vi "Read.vi"(7 "Read Type":T1, 8 "error in (no error)":errorcluster, 11 "NetworkStreamReader in":refnum<class "NetworkStreamReader.lvclass">) -> (0 "error out":errorcluster, 2 "element":variant, 3 "NetworkStreamReader out":refnum<class "NetworkStreamReader.lvclass">)   [LabVIEW 2011, in "NetworkStreamReader.lvclass"]
doc: "Returns the requested value (either the next element available in the buffer or the most recent element). If there are no elements available in the queue, this VI will return the last valid value it returned."
uses:
  NetworkStreamReader.lvclass
  readType.ctl
  NetworkStreamReader.lvclass/NetworkStreamReader.ctl
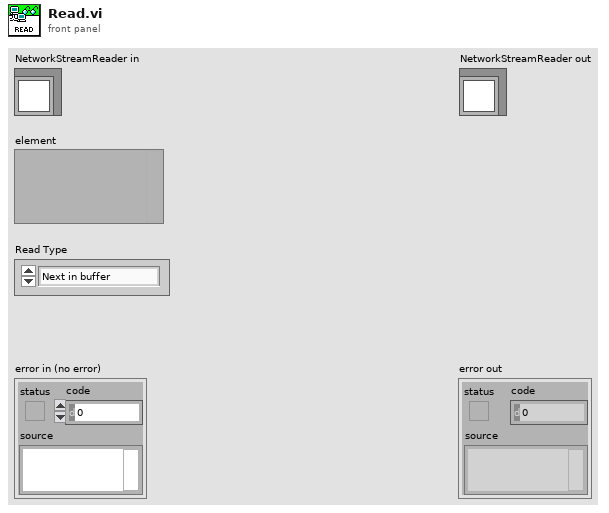
[diagram p1: front panel]
types:
  T1 = typedef "NetworkStreamReader.lvclass/readType.ctl" = enum16{"Next in buffer", "Most current"}
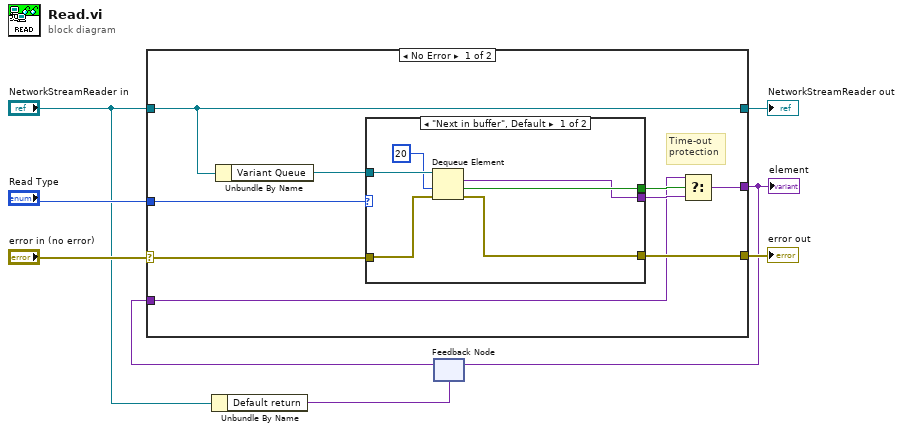
[diagram p0: block diagram]
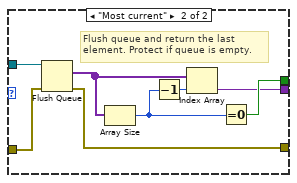
[diagram p2: hidden frame]
diagram:
  n1 = Unbundle By Name("NetworkStreamReader in") -> ("Default return"=w1:variant)
  n2 = feedback #1(w1) -> (w4:variant)
  n3 = case shown="No Error" "error in (no error)" {
    selector: "error in (no error)" -> [w14 w33]
    tunnel: [w15 w33] -> w7
    tunnel: [w17 w32] -> w6
    tunnel: "NetworkStreamReader in" -> [w17 w32]
    tunnel: [w9 _] -> w5
    tunnel: w4 -> [w10 _]
    tunnel: "Read Type" -> [w13 _]
    frame No Error {
      # "Time-out \nprotection"
      n4 = Unbundle By Name(w17) -> ("Variant Queue"=w16:refnum<queue>)
      n5 = case shown="\"Next in buffer\", Default" w13 {
        tunnel: w16 -> [w23 w31]
        tunnel: [w18 w28] -> w15
        tunnel: w14 -> [w21 w30]
        tunnel: [w20 w29] -> w12
        tunnel: [w19 w24] -> w11
        frame "Next in buffer", Default {
          n6 = Dequeue Element(queue=w23, timeout in ms (-1)=20, error in (no error)=w21) -> (element=w19:variant, timed out?=w20:bool, error out=w18:errorcluster)  [unwired: 1 out]
        }
        frame "Most current" {
          # "Flush queue and return the last\nelement. Protect if queue is empty."
          n7 = Flush Queue(queue=w31, error in (no error)=w30) -> (remaining elements=w26:variant[], error out=w28:errorcluster)  [unwired: 1 out]
          n8 = Array Size(array=w26) -> (size(s)=w27:i32)
          n9 = Decrement(x=w27) -> (x-1=w25:i32)
          n10 = Index Array(array=w26, index=w25) -> (element=w24:variant)
          n11 = Equal To 0?(x=w27) -> (x = 0?=w29:bool)
        }
      }
      n12 = Select(t=w10, s=w12, f=w11) -> (s? t:f=w9:variant)
    }
    frame Error {
    }
  }
  "error out" <- w7
  "NetworkStreamReader out" <- w6
  "element" <- w5
  n13 = feedback-in #1(w5) -> ()
